vi "ke37xx Error Query (Multiple).vi"(0 "VISA resource name":refnum<visa-resource-name>, 11 "error in (no error)":errorcluster) -> (4 "VISA resource name out":refnum<visa-resource-name>, 8 "Error":i32[](array[numeric]), 10 "Error Message":string, 15 "error out":errorcluster)   [LabVIEW 2009, in "Keithley 3700 Series.lvlib"]
doc: "This VI reads the error queue from the instrument. It continues to read from the error queue until it reads a 0, \"No error\". If the instrument does not support an error query, a warning is returned."
uses:
  <instrlib>/Keithley 3706/Keithley 3700 Series.lvlib
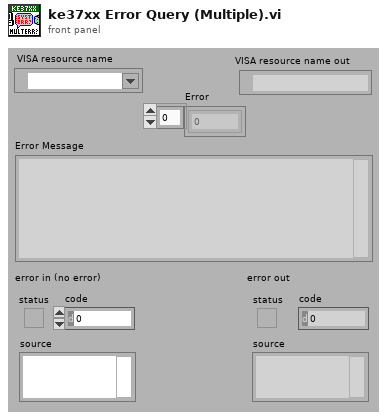
[diagram p1: front panel]
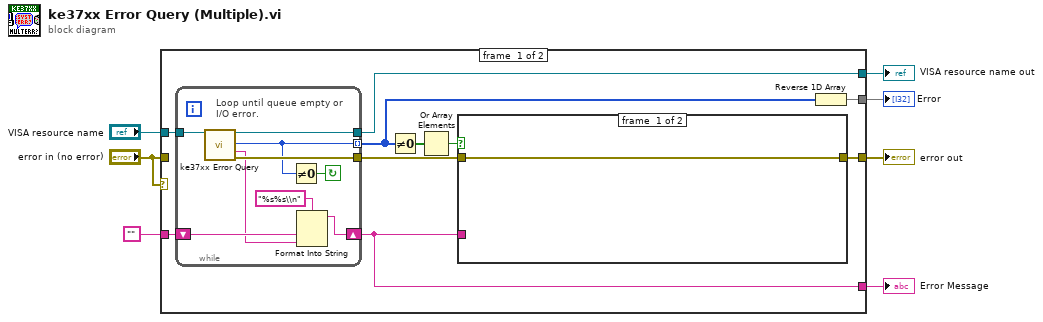
[diagram p0: block diagram]
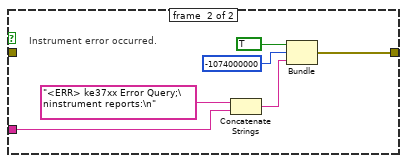
[diagram p2: hidden frame]
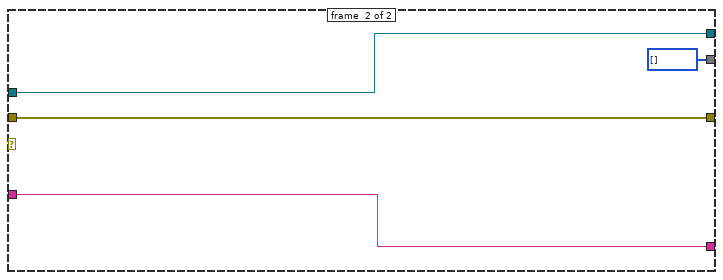
[diagram p3: hidden frame]
diagram:
  n1 = case shown="No Error" "error in (no error)" {
    tunnel: "" -> [w17 w36]
    tunnel: [w16 w37] -> w6
    tunnel: "VISA resource name" -> [w15 w35]
    tunnel: [w14 w35] -> w4
    tunnel: "error in (no error)" -> [_ w37]
    tunnel: [w13 i32[] []] -> w3
    tunnel: [w12 w36] -> w2
    frame #0 {
      n2 = while {
        tunnel: [w19] -> w11 mode=indexing
        shift-left: w17 -> [w22]
        shift-right: [w20] -> w12
        tunnel: w15 -> [w24]
        tunnel: [w26] -> w14
        tunnel: [w23] -> w8
        stop <- w25 continue-if-true
        # "Loop until queue empty or I/O error."
        n3 = call <instrlib>:"ke37xx Error Query.vi"("VISA resource name"=w24) -> ("VISA resource name out"=w26:refnum<visa-resource-name>, "Error"=w19:i32, "Error Message"=w18:string, "error out"=w23:errorcluster)  [unwired: 1 in, 10 out]
        n4 = Not Equal To 0?(x=w19) -> (x != 0?=w25:bool)
        n5 = Format Into String(format string="%s%s\\n", w22, w18) -> (resulting string=w20:string)  [unwired: 2 in, 1 out]
      }
      n6 = Not Equal To 0?(x=w11) -> (x != 0?=w10:bool[])
      n7 = Or Array Elements(Boolean array=w10) -> (logical OR=w9:bool)
      n8 = case shown="False" w9 {
        tunnel: [w27 w28] -> w16
        tunnel: w12 -> [_ w33]
        tunnel: w8 -> [w27 _]
        frame #0 {
        }
        frame #1 {
          # "Instrument error occurred."
          n9 = Concatenate Strings("<ERR> ke37xx Error Query;\ninstrument reports:\n" ("Source"), w33) -> (w30:string)
          n10 = Bundle("Status"=TRUE, "Error"=-1074000000, w30) -> (w28:cluster{"Status":bool, "Error":i32, string})  [unwired: 1 out]
        }
      }
      n11 = Reverse 1D Array(array=w11) -> (reversed array=w13:i32[])
    }
    frame #1 {
    }
  }
  "Error Message" <- w2
  "error out" <- w6
  "VISA resource name out" <- w4
  "Error" <- w3
